vi "Process.vi"(8 "error in":errorcluster, 11 "Transport":refnum<class "SMO.Transport.lvclass">) -> (0 "error out":errorcluster, 3 "Transport out":refnum<class "SMO.Transport.lvclass">)   [LabVIEW 2019, in "SMO.Transport.lvclass"]
doc: "---------------------------------------------------------------\nJKI State Machine Objects™\nhttp://jki.net/state-machine-objects/\nCopyright (C) 2005-2015, JKI <info@jki.net>\nALL RIGHTS RESERVED"
uses:
  SMO.Transport.lvclass
  C:/Program Files (x86)/National Instruments/LabVIEW 2019/vi.lib/JKI/JKI SMO/SMO/SMO.lvclass
  SMO.Transport.lvclass/SMO.Transport.ctl
  Transport/Transport.lvclass/Transport.ctl
  <vilib>/JKI/JKI SMO/SMO/SMO.lvclass/SMO.ctl
  <userlib>/LevyLab/Instrument Framework/Instrument Types/Cryostat/Typedefs/Magnet Axis--Enum.ctl
  <userlib>/LevyLab/Instrument Framework/Instrument Types/Cryostat/Typedefs/Magnet Mode--Enum.ctl
  <userlib>/LevyLab/Lockin-Multichannel/Instrument.DAQ/Typedefs/Sweep.Configuration--Cluster.ctl
  <userlib>/LevyLab/Lockin-Multichannel/Instrument.DAQ/Typedefs/Sweep.Channel--Cluster--Array.ctl
  <userlib>/LevyLab/Lockin-Multichannel/Instrument.DAQ/Typedefs/Sweep.Channel--Cluster.ctl
  <userlib>/LevyLab/Lockin-Multichannel/Instrument.DAQ/Typedefs/Sweep.Pattern--Enum.ctl
  <vilib>/JKI/JKI SMO/SMO/Private/ReftoDVR--SMO.vi
  Control Experiment/Control Experiment.lvclass
  <vilib>/JKI/JKI SMO/SMO/SMO.lvclass
  <userlib>/LevyLab/Instrument Framework/Instrument Types/Cryostat/Instrument.Cryostat.lvclass
  <userlib>/LevyLab/Instrument Framework/Instrument Types/Strain/Instrument.Strain.lvclass
  <userlib>/LevyLab/Instrument Framework/Instrument Types/Delay Line/Instrument.DelayLine.lvclass
  <userlib>/LevyLab/Instrument Framework/Instrument Types/CBridge/Instrument.CBridge.lvclass
  <userlib>/LevyLab/Lockin-Multichannel/Instrument.Lockin/Instrument.Lockin.lvclass
  Transport/Transport.lvclass
  <userlib>/LevyLab/Lockin-Multichannel/Instrument.DAQ/Instrument.DAQ.lvclass
panel:
  # "For instructions on how to use the JKI State Machine Objects, examples and video tutorials, visit:\nhttp://jki.net/state-machine-objects/\n\nJKI State Machine Objects™\nhttp://jki.net/state-machine-objects/\nCopyright (C) 2005-2015, JKI <info@jki.net>\nALL RIGHTS RESERVED"
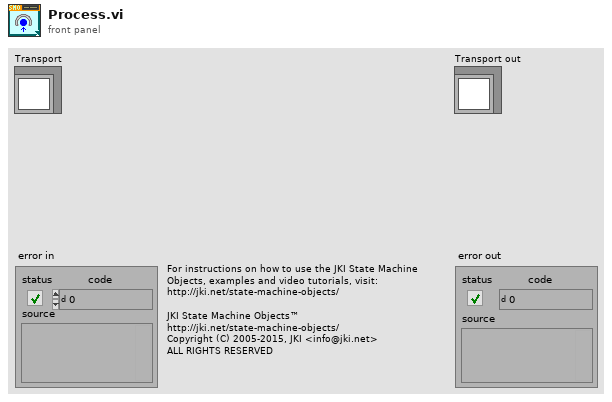
[diagram p1: front panel]
types:
  T1 = enum32{"invalid app kind", "Development System", "Run Time System", "Student Edition", "Embedded LabVIEW", "Evaluation", "Custom"}
  T2 = enum32{"Invalid", "Standard", "Closed", "Hidden", "Minimized", "Maximized"}
  T3 = enum32{"Bad", "Idle", "Run top level", "Running"}
  T4 = typedef "Instrument.Cryostat.lvclass/Magnet Mode--Enum.ctl" = enum16{"Persistent", "Driven"}
  T5 = typedef "Instrument.Cryostat.lvclass/Magnet Axis--Enum.ctl" = enum16{"Z", "X", "Y"}
  T6 = typedef "Instrument.DAQ.lvclass/Sweep.Configuration--Cluster.ctl" = cluster{"Sweep Time (s)":dbl, "Initial Wait (s)":dbl, "Return to Start":bool, "Channels":T7}
  T7 = typedef "Instrument.DAQ.lvclass/Sweep.Channel--Cluster--Array.ctl" = T8[]
  T8 = typedef "Instrument.DAQ.lvclass/Sweep.Channel--Cluster.ctl" = cluster{"Enable?":bool, "Channel":u16, "Start":dbl, "End":dbl, "Pattern":T9, "Table":dbl[]}
  T9 = typedef "Instrument.DAQ.lvclass/Sweep.Pattern--Enum.ctl" = enum16{"Ramp /", "Ramp /\\", "Smooth Ramp _/", "Smooth Ramp _/\\_", "Table"}
  T10 = typedef "Control Experiment.lvclass/Instruments--cluster.ctl" = cluster{"KH7008":refnum<class "Instrument.KH7008.lvclass">[], "Lockin":refnum<class "Instrument.Lockin.lvclass">, "Temperature":refnum<class "Instrument.Cryostat.lvclass">, "Magnet":refnum<class "Instrument.Cryostat.lvclass">, "Rotator":refnum<class "Instrument.Cryostat.lvclass">, "Level":refnum<class "Instrument.Cryostat.lvclass">, "Capacitance Bridge":refnum<class "Instrument.CBridge.lvclass">, "Delay Line":refnum<class "Instrument.DelayLine.lvclass">, "Strain Cell":refnum<class "Instrument.Strain.lvclass">, "VNA":refnum<class "Instrument.VNA.lvclass">, "Voltage Source":refnum<class "Instrument.VSource.lvclass">}
  T11 = cluster{"Core":cluster{"Current VI Reference":refnum<vi>, "Close Panel on Exit?":bool, "error":errorcluster}, "Self Reference":refnum<class "SMO.Transport.lvclass">, "C.E.":refnum<class "Control Experiment.lvclass">, "Instruments":T10, "value":variant, "wait":bool}
  T12 = cluster{"Current VI Reference":refnum<vi>, "Close Panel on Exit?":bool, "error":errorcluster}
  T13 = typedef "SMO.lvclass/Protected Events.ctl" = cluster{"StopProcesses":refnum<user-event>, "AbortProcesses":refnum<user-event>, "Config Changed":refnum<user-event>, "Dependency":refnum<user-event>}
  T14 = typedef "SMO.Transport.lvclass/PrivateEvents--Cluster.ctl" = cluster{"Configure":refnum<user-event>}
  T15 = typedef "Instrument.DAQ.lvclass/Get State-enum.ctl" = enum16{"idle", "created", "started", "stopped", "sweeping"}
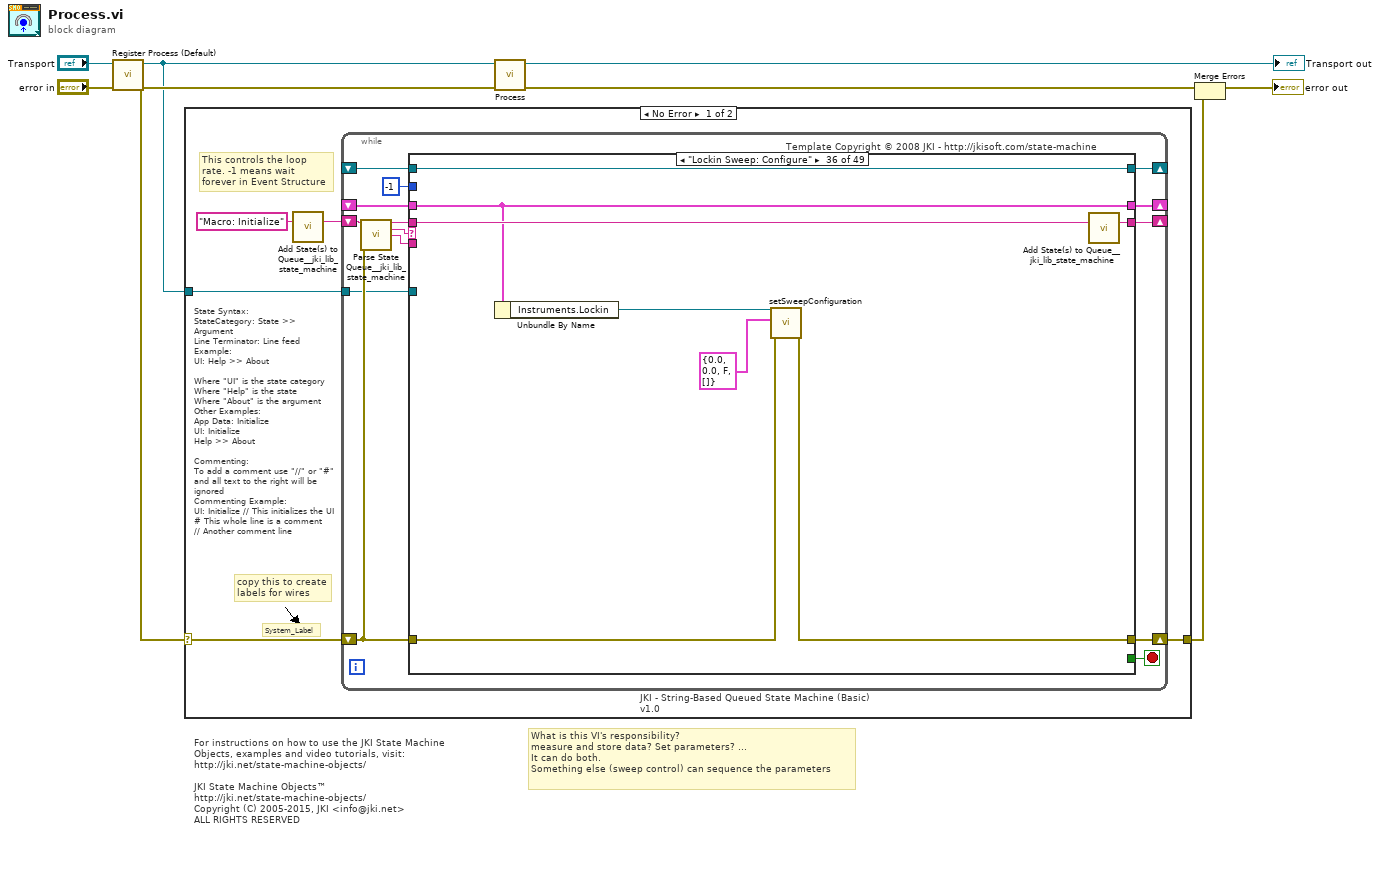
[diagram p0: block diagram]
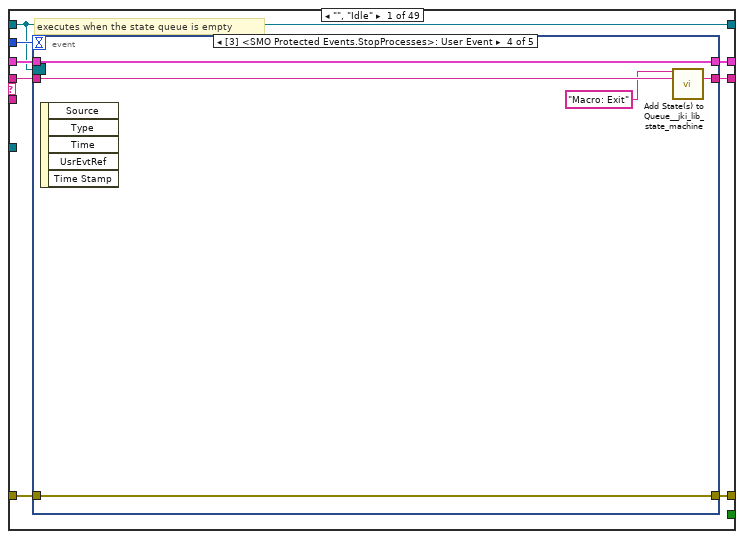
[diagram p2: hidden frame]
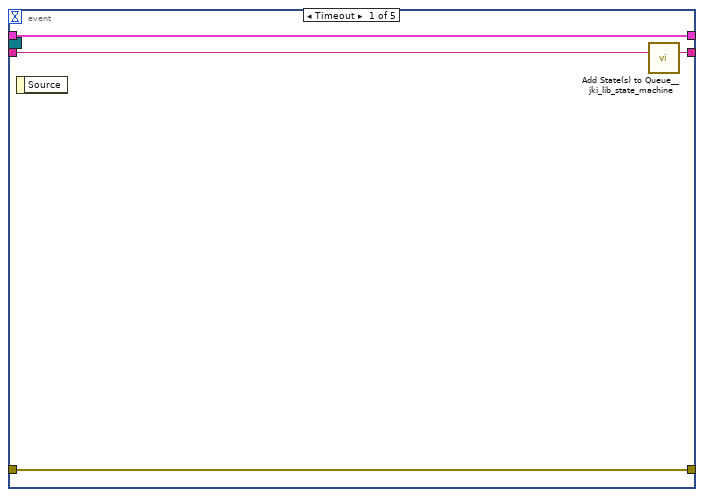
[diagram p3: hidden frame]
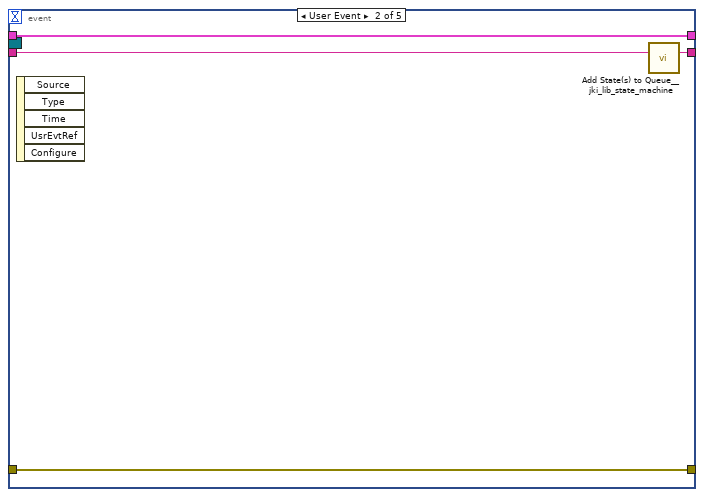
[diagram p4: hidden frame]
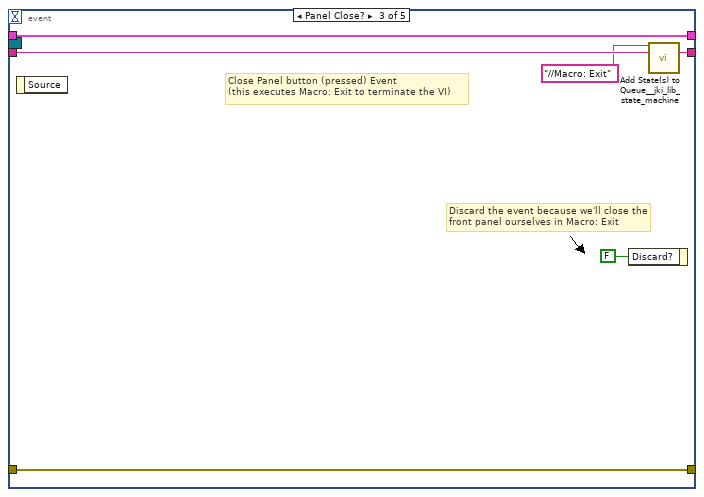
[diagram p5: hidden frame]
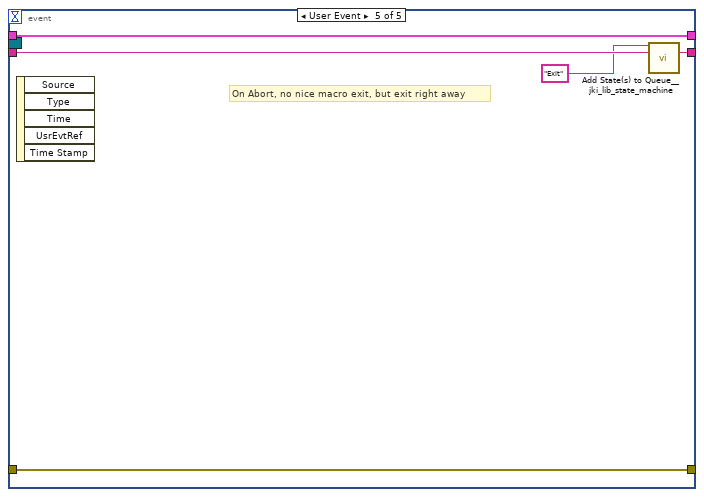
[diagram p6: hidden frame]
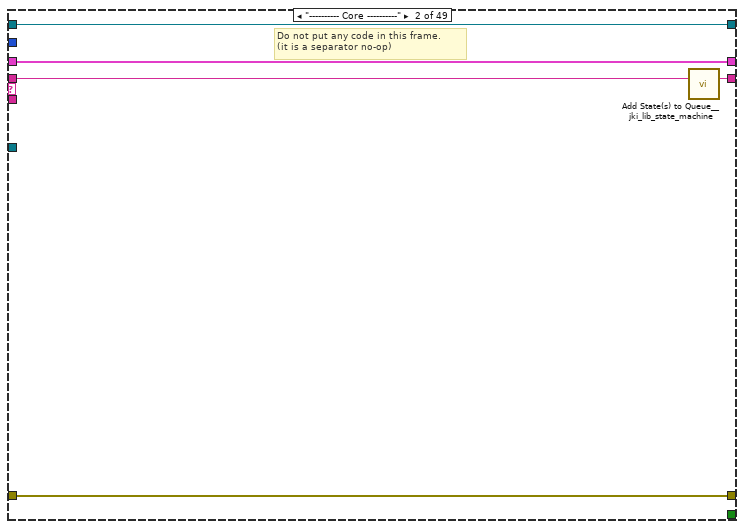
[diagram p7: hidden frame]
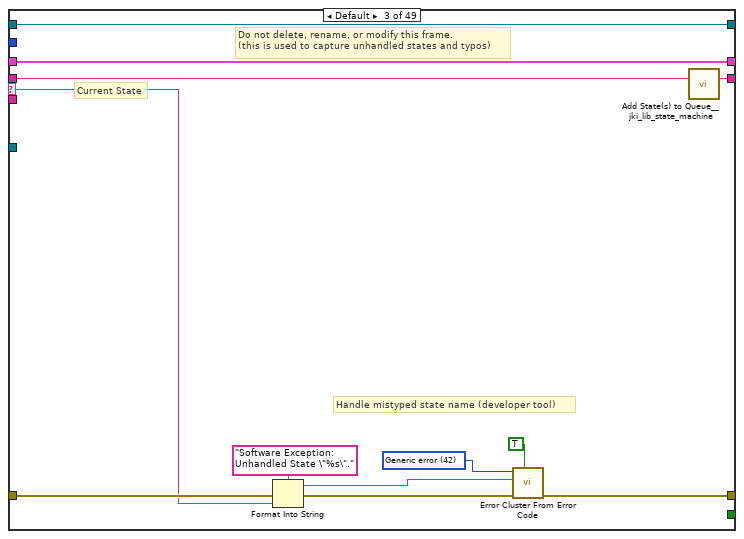
[diagram p8: hidden frame]
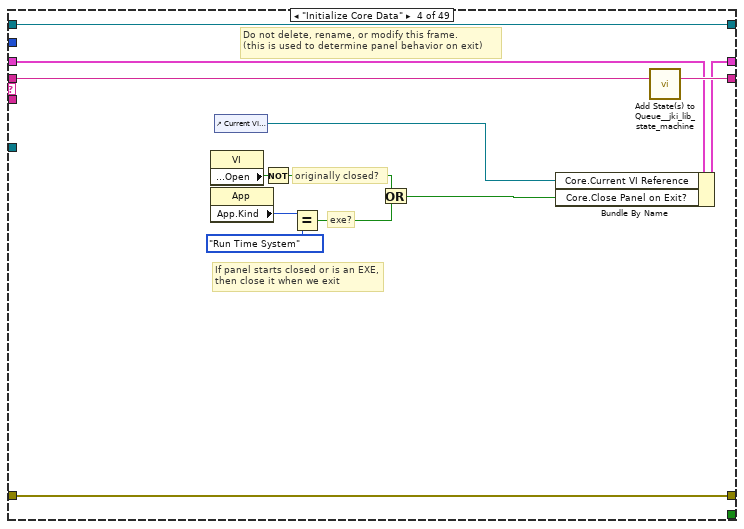
[diagram p9: hidden frame]
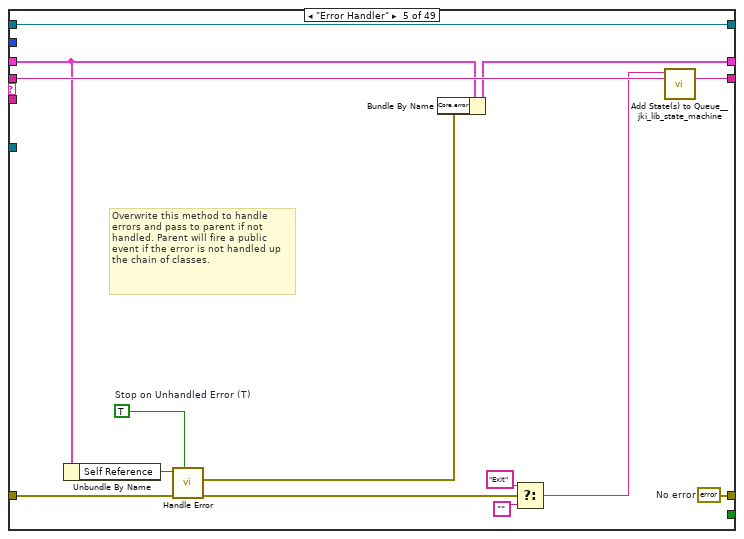
[diagram p10: hidden frame]
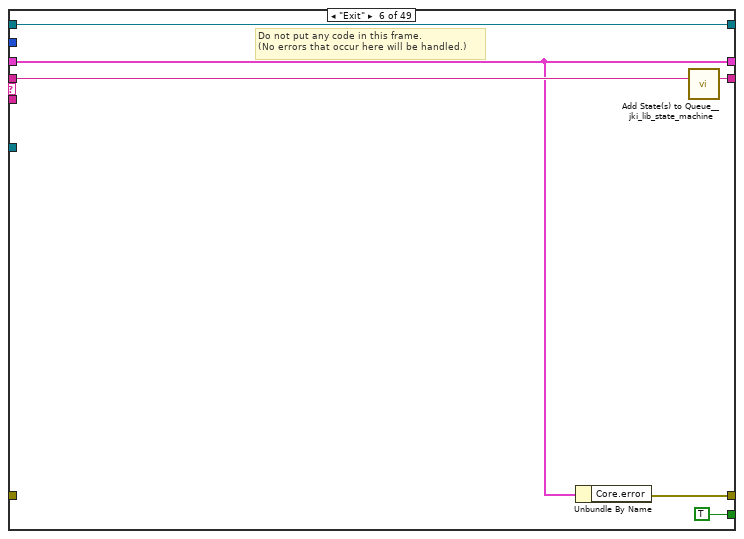
[diagram p11: hidden frame]
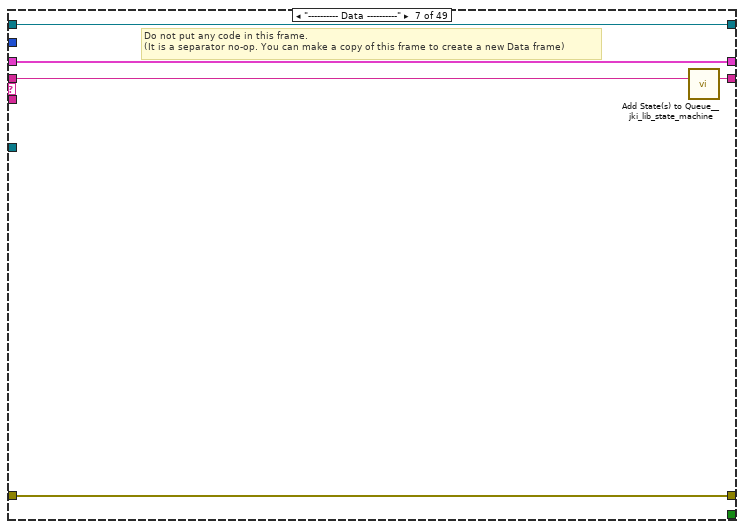
[diagram p12: hidden frame]
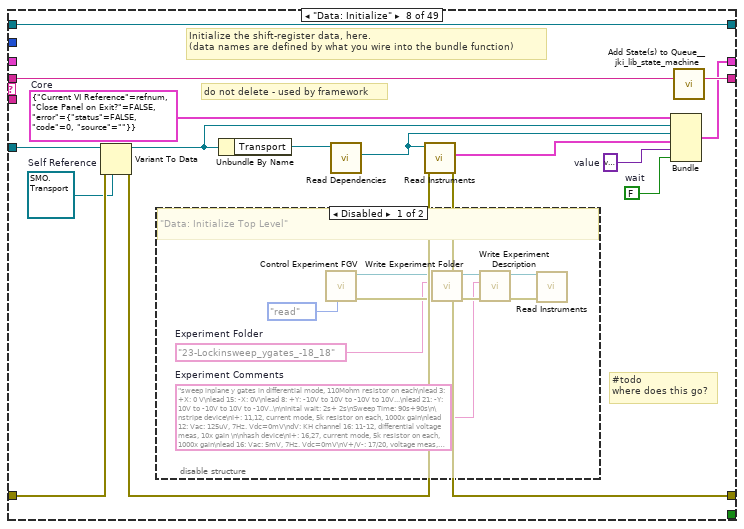
[diagram p13: hidden frame]
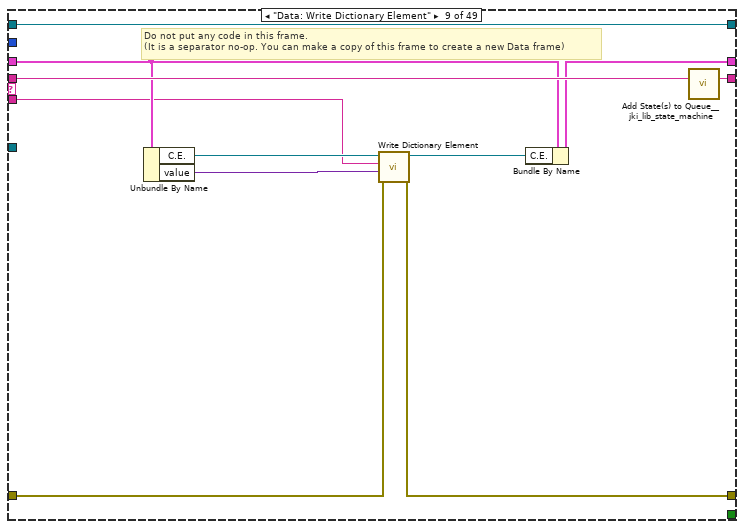
[diagram p15: hidden frame]
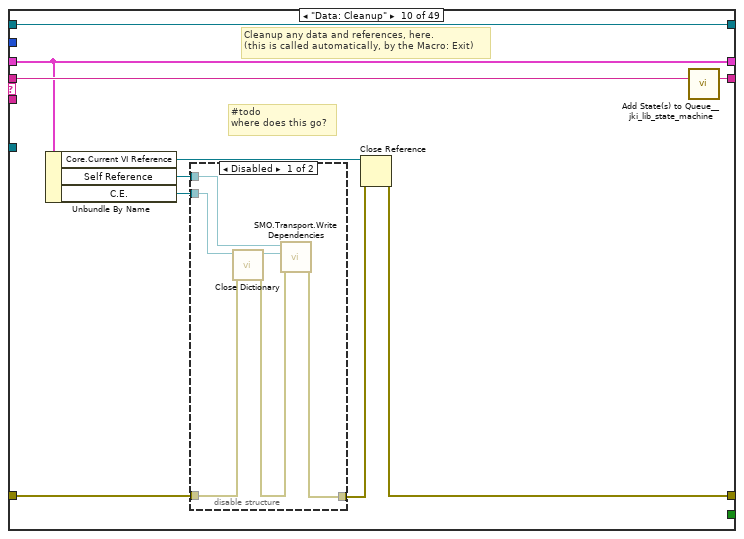
[diagram p16: hidden frame]
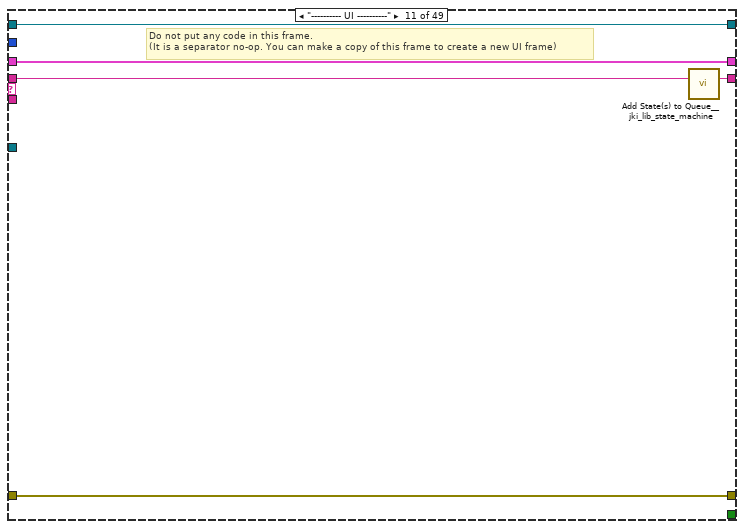
[diagram p18: hidden frame]
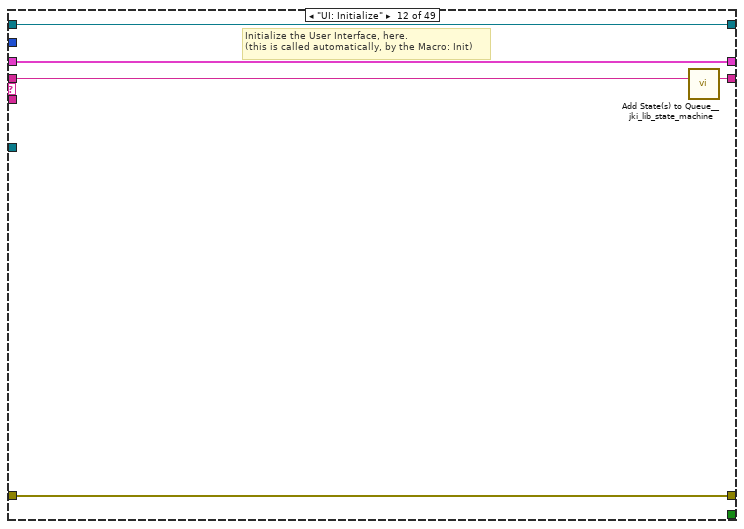
[diagram p19: hidden frame]
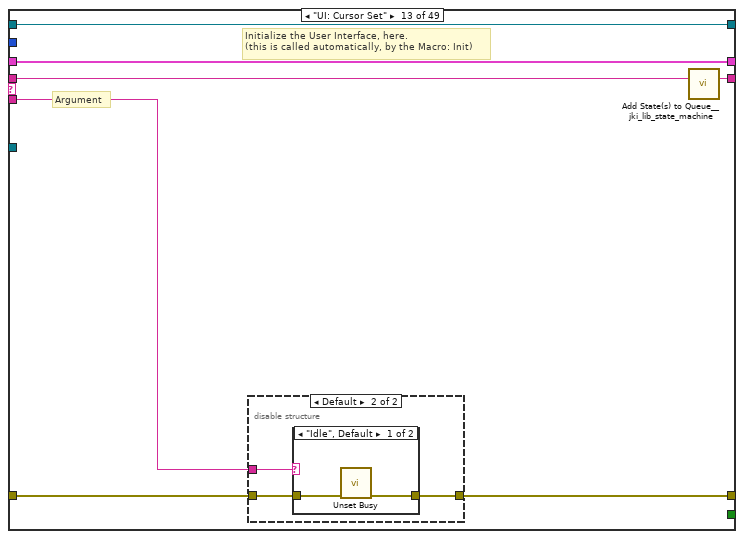
[diagram p20: hidden frame]
diagram:
  # "What is this VI's responsibility?\nmeasure and store data? Set parameters? ...\nIt can do both.\nSomething else (sweep control) can sequence the parameters"
  # "For instructions on how to use the JKI State Machine Objects, examples and video tutorials, visit:\nhttp://jki.net/state-machine-objects/\n\nJKI State Machine Objects™\nhttp://jki.net/state-machine-objects/\nCopyright (C) 2005-2015, JKI <info@jki.net>\nALL RIGHTS RESERVED"
  n1 = call <vilib>:"Register Process (Default).vi"("error in (no error)"="error in", "SMO"="Transport") -> ("error out"=w5:errorcluster, "SelfRef"=w4:refnum<class "SMO.Transport.lvclass">)  [unwired: 8 in]
  n2 = case shown="No Error" w5 {
    selector: w5 -> [w10 w561]
    tunnel: w4 -> [w11 _]
    tunnel: [w9 w561] -> w1
    frame No Error {
      # "State Syntax:\nStateCategory: State >> Argument\nLine Terminator: Line feed\nExample:\nUI: Help >> About\n\nWhere \"UI\" is the state category\nWhere \"Help\" is the state\nWhere \"About\" is the argument\nOther Examples:\nApp Data: Initialize\nUI: Initialize\nHelp >> About\n\nCommenting:\nTo add a comment use \"//\" or \"#\" and all text to the right will be ignored\nCommenting Example:\nUI: Initialize // This initializes the UI\n# This whole line is a comment\n// Another comment line"
      # "copy this to create labels for wires"
      # "This controls the loop rate. -1 means wait forever in Event Structure"
      # "System_Label"
      n3 = call <vilib>:"Add State(s) to Queue__jki_lib_state_machine.vi"("State(s) in (\"\")"="Macro: Initialize") -> ("States Out"=w13:string)  [unwired: 14 in]
      n4 = while "JKI - String-Based Queued State Machine (Basic) v1.0" {
        shift-right: [w20] -> _
        shift-left: _ -> [w19]
        shift-right: [w23] -> w9
        shift-left: w10 -> [w17]
        shift-right: [w22] -> _
        shift-left: w13 -> [w24]
        tunnel: w11 -> [w16]
        shift-right: [w15] -> _
        shift-left: _ -> [w14]
        stop <- w21 stop-if-true
        # "Template Copyright © 2008 JKI - http://jkisoft.com/state-machine"
        n5 = call <vilib>:"Parse State Queue__jki_lib_state_machine.vi"("State Queue"=w24, "Error In (no error)"=w17) -> ("Remaining States"=w26:string, "Current State"=w27:string, "Arguments"=w25:string)  [unwired: 11 in]
        n6 = case shown="\"Lockin Sweep: Configure\"" w27 {
          selector: w27 -> [_ _ w66 _ _ _ _ _ _ _ _ _ _ _ _ _ _ _ _ _ _ _ _ _ w312 _ _ _ _ _ _ _ _ _ _ _ _ _ _ _ _ _ _ _ _ _ _ _ _]
          tunnel: w26 -> [w35 w64 w70 w89 w103 w109 w114 w130 w150 w160 w172 w177 w184 w200 w232 w246 w251 w265 w270 w281 w286 w298 w304 w309 w324 w334 w348 w362 w374 w386 w398 w410 w422 w434 w441 w449 w458 w467 w475 w480 w488 w497 w506 w515 w524 w533 w542 w551 w560]
          tunnel: w25 -> [_ _ _ _ _ _ _ _ w140 _ _ _ w178 w194 _ _ _ _ _ _ _ _ _ _ w313 w325 w343 w357 w369 w381 w393 w405 w417 w429 _ _ _ _ _ _ _ _ _ _ _ _ _ _ _]
          tunnel: w19 -> [w33 w61 w68 w80 w97 w105 w111 _ w145 w151 w169 w175 w182 w196 w229 w242 w248 w256 w267 w278 w283 w296 w302 w306 w320 w330 w344 w358 w370 w382 w394 w406 w418 w430 w438 w446 w455 w464 w472 w478 w485 w491 w500 w509 w518 w527 w536 w545 w554]
          tunnel: [w32 w62 w72 w86 w98 w104 w112 w119 w142 w157 w170 w174 w179 w197 w230 w244 w249 w263 w268 w272 w284 w292 w300 w307 w322 w331 w345 w359 w371 w383 w395 w407 w419 w431 w439 w443 w450 w459 w469 w476 w482 w493 w502 w511 w520 w529 w538 w547 w556] -> w23
          tunnel: w17 -> [w31 w62 w71 w86 w99 _ w112 w127 w143 w153 w170 w174 w180 w198 w230 w244 w249 w263 w268 w273 w284 w293 w300 w307 w322 w326 w337 w353 w365 w377 w389 w401 w413 w425 w439 w444 w453 w462 w470 w476 w482 w489 w498 w507 w516 w525 w534 w543 w552]
          tunnel: [w34 w63 w69 w88 w102 w108 w113 w129 w149 w159 w171 w176 w183 w199 w231 w245 w250 w264 w269 w280 w285 w297 w303 w308 w323 w333 w347 w361 w373 w385 w397 w409 w421 w433 w440 w448 w457 w466 w474 w479 w487 w496 w505 w514 w523 w532 w541 w550 w559] -> w22
          tunnel: [_ _ _ _ _ TRUE _ _ _ _ _ _ _ _ _ _ _ _ _ _ _ _ _ _ _ _ _ _ _ _ _ _ _ _ _ _ _ _ _ _ _ _ _ _ _ _ _ _ _] -> w21
          tunnel: [w30 w61 w68 w87 w96 w105 w111 w128 w144 w151 w169 w175 w182 w196 w229 w242 w248 w256 w267 w278 w283 w296 w302 w306 w319 w330 w344 w358 w370 w382 w394 w406 w418 w430 w438 w446 w455 w464 w472 w478 w484 w494 w503 w512 w521 w530 w539 w548 w557] -> w20
          tunnel: -1 ("Timeout") -> [w29 _ _ _ _ _ _ _ _ _ _ _ _ _ _ _ _ _ _ _ _ _ _ _ _ _ _ _ _ _ _ _ _ _ _ _ _ _ _ _ _ _ _ _ _ _ _ _ _]
          tunnel: w16 -> [_ _ _ _ _ _ _ w126 _ _ _ _ _ _ _ _ _ _ _ _ _ _ _ _ _ _ _ _ _ _ _ _ _ _ _ _ _ _ _ _ _ _ _ _ _ _ _ _ _]
          tunnel: [w28 w60 w65 w77 w101 w106 w110 w125 w148 w156 w168 w173 w181 w193 w228 w243 w247 w257 w266 w279 w282 w295 w301 w305 w321 w332 w346 w360 w372 w384 w396 w408 w420 w432 w437 w447 w456 w465 w473 w477 w486 w495 w504 w513 w522 w531 w540 w549 w558] -> w15
          tunnel: w14 -> [w28 w60 w65 w77 w101 w106 w110 w125 w148 w156 w168 w173 w181 w193 w228 w243 w247 w257 w266 w279 w282 _ w301 w305 w321 w332 w346 w360 w372 w384 w396 w408 w420 w432 w437 w447 w456 w465 w473 w477 w486 w495 w504 w513 w522 w531 w540 w549 w558]
          frame "", "Idle" {
            # "executes when the state queue is empty"
            n7 = event shown="[3] <SMO Protected Events.StopProcesses>: User Event" {
              selector: w28 -> [_ _ _ _ _]
              dyn-events: _ -> [_ _ _ _ _]
              timeout: w29 -> [_ _ _ _ _]
              tunnel: w35 -> [w39 w43 w49 w54 w59]
              tunnel: [w38 w42 w48 w53 w58] -> w34
              tunnel: w33 -> [w37 w41 w46 w51 w56]
              tunnel: [w36 w40 w47 w52 w57] -> w32
              tunnel: w31 -> [w36 w40 w47 w52 w57]
              tunnel: [w37 w41 w46 w51 w56] -> w30
              event Timeout {
                n8 = event-data() -> ()  [unwired: 1 in, 1 out]
                n9 = call <vilib>:"Add State(s) to Queue__jki_lib_state_machine.vi"("State(s) in (\"\")"=w39) -> ("States Out"=w38:string)  [unwired: 14 in]
              }
              event User Event {
                n10 = event-data() -> ()  [unwired: 1 in, 5 out]
                n11 = call <vilib>:"Add State(s) to Queue__jki_lib_state_machine.vi"("State(s) in (\"\")"=w43) -> ("States Out"=w42:string)  [unwired: 14 in]
              }
              event Panel Close? {
                # "Discard the event because we'll close the front panel ourselves in Macro: Exit"
                # "Close Panel button (pressed) Event\n(this executes Macro: Exit to terminate the VI)"
                n12 = event-data() -> ()  [unwired: 1 in, 1 out]
                n13 = event-data("Discard?"=FALSE) -> ()  [unwired: 1 in, 1 out]
                n14 = call <vilib>:"Add State(s) to Queue__jki_lib_state_machine.vi"("State(s) in Front (\"\")"="//Macro: Exit", "State(s) in (\"\")"=w49) -> ("States Out"=w48:string)  [unwired: 13 in]
              }
              event User Event {
                n15 = event-data() -> ()  [unwired: 1 in, 5 out]
                n16 = call <vilib>:"Add State(s) to Queue__jki_lib_state_machine.vi"("State(s) in Front (\"\")"="Macro: Exit", "State(s) in (\"\")"=w54) -> ("States Out"=w53:string)  [unwired: 13 in]
              }
              event User Event {
                # "On Abort, no nice macro exit, but exit right away"
                n17 = event-data() -> ()  [unwired: 1 in, 5 out]
                n18 = call <vilib>:"Add State(s) to Queue__jki_lib_state_machine.vi"("State(s) in Front (\"\")"="Exit", "State(s) in (\"\")"=w59) -> ("States Out"=w58:string)  [unwired: 13 in]
              }
            }
          }
          frame "---------- Core ----------" {
            # "Do not put any code in this frame.\n(it is a separator no-op)"
            n19 = call <vilib>:"Add State(s) to Queue__jki_lib_state_machine.vi"("State(s) in (\"\")"=w64) -> ("States Out"=w63:string)  [unwired: 14 in]
          }
          frame Default {
            w75 = 42 items=["No error", "Argument error", "Memory is full", "Out of zone", "End of file", "File already open", "Generic file I/O error", "File not found", "File permission error", "Disk is full", "Duplicate path", "Too many files open", "System feature not enabled", "Resource file not found", "Cannot add resource", "Resource not found", "Image not found", "Image memory error", "Pen does not exist", "Config type invalid", "Config token not found", "Config parse error", "Config memory error", "Bad external code format", "Bad external code offset", "External code not present", "Null window", "Destroy window error", "Null menu", "Print aborted", "Bad print record", "Print driver error", "Windows error during printing", "Memory error during printing", "Print dialog error", "Generic print error", "Invalid device refnum", "Device not found", "Device parameter error", "Device unit error", "Cannot open device", "Device call aborted", "Generic error", "Cancelled by user", "Object ID too low", "Object ID too high", "Object not in heap", "Unknown heap", "Unknown object (invalid DefProc)", "Unknown object (DefProc not in table)", "Message out of range", "Invalid (null) method", "Unknown message", "Manager call not supported", "Bad address", "Network operation in progress", "Network operation timed out", "Connection is busy", "Network attribute not supported", "Network error", "Address in use", "System out of memory", "Connection aborted", "Connection refused", "Not connected", "Already connected", "Connection closed", "Initialization error (interapplication manager)", "Bad occurrence", "Wait on unbound occurrence handler", "Occurrence queue overflow", "Datalog type conflict", "Unused", "Unrecognized type (interapplication manager)", "Memory corrupt", "Failed to make temporary DLL", "Old CIN version", "Drag socket not found", "Failed to load drop-object", "Failed to register OLE object", "Failed to release OLE object", "Format specifier type mismatch", "Unknown format specifier", "Too few format specifiers", "Too many format specifiers", "Scan failed", "Newer CIN version", "Error converting to variant", "Runtime menu error", "Password tampered", "Variant attribute not found", "Incompatible variant data type", "Event data is not available", "Event Store is not present", "Occurrence is not found", "Event Queue is not created", "Event info is not available", "Refnum passed is NULL", "Error retrieving Class GUID", "Error retrieving CoClass GUID", "Error retrieving TypeLib GUID.", "Bad built application magic bytes.", "Specific driver is different from the specific driver associated with the Logical Name.", "There is no session opened to the class driver.", "Max Error", "MAX - Error with config objects", "MAX - Error loading configuration", "MAX - Group not supported"]
            # "Current State"
            # "Do not delete, rename, or modify this frame.\n(this is used to capture unhandled states and typos)"
            # "Handle mistyped state name (developer tool)"
            n20 = Format Into String(format string="Software Exception: Unhandled State \"%s\"." ("message"), error in=w71, w66) -> (resulting string=w74:string, error out=w73:errorcluster)  [unwired: 1 in]
            n21 = call <vilib>:"Error Cluster From Error Code.vi"("show call chain? (False)"=TRUE, "error in (no error)"=w73, "error message (\"\")"=w74, "error code (0)"=w75) -> ("error out"=w72:errorcluster)  [unwired: 5 in]
            n22 = call <vilib>:"Add State(s) to Queue__jki_lib_state_machine.vi"("State(s) in (\"\")"=w70) -> ("States Out"=w69:string)  [unwired: 14 in]
          }
          frame "Initialize Core Data" {
            # "Do not delete, rename, or modify this frame.\n(this is used to determine panel behavior on exit)"
            # "originally closed?"
            # "exe?"
            # "If panel starts closed or is an EXE, then close it when we exit"
            n23 = property class="VI"() -> ("Front Panel.Open"=w85:bool)  [unwired: 2 in, 2 out]
            n24 = property class="App"() -> ("App.Kind"=w84:T1)  [unwired: 2 in, 2 out]
            n25 = control-ref of="Current VI Reference"() -> (w78:refnum<vi>)
            n26 = Not(x=w85) -> (.not. x?=w82:bool)
            n27 = Equal?(x=w84, y=T1."Run Time System" ("Application:Kind")) -> (x = y?=w81:bool)
            n28 = Or(x=w82, y=w81) -> (x .or. y?=w79:bool)
            n29 = Bundle By Name(cluster=w80, "Core.Current VI Reference"=w78, "Core.Close Panel on Exit?"=w79) -> (w87:T11)
            n30 = call <vilib>:"Add State(s) to Queue__jki_lib_state_machine.vi"("State(s) in (\"\")"=w89) -> ("States Out"=w88:string)  [unwired: 14 in]
          }
          frame "Error Handler" {
            w90 = TRUE  # Stop on Unhandled Error (T)
            w98 = errorcluster {"status"=FALSE, "code"=0, "source"=""}  # No error
            # "Overwrite this method to handle errors and pass to parent if not handled. Parent will fire a public event if the error is not handled up the chain of classes."
            n31 = Unbundle By Name(w97) -> ("Self Reference"=w100:refnum<class "SMO.Transport.lvclass">)
            n32 = call-dynamic "Handle Error.vi"("Stop on Unhandled Error (T)"=w90, "error in"=w99, "SMO"=w100) -> ("handling error"=w91:errorcluster, "Unhandled error"=w94:errorcluster)  [unwired: 6 in, 1 out]
            n33 = Bundle By Name(cluster=w97, "Core.error"=w94) -> (w96:T11)
            n34 = Select(t="Exit", s=w91, f="") -> (s? t:f=w95:string)
            n35 = call <vilib>:"Add State(s) to Queue__jki_lib_state_machine.vi"("State(s) in Front (\"\")"=w95, "State(s) in (\"\")"=w103) -> ("States Out"=w102:string)  [unwired: 13 in]
          }
          frame "Exit" {
            # "Do not put any code in this frame.\n(No errors that occur here will be handled.)"
            n36 = Unbundle By Name(w105) -> ("Core.error"=w104:errorcluster)
            n37 = call <vilib>:"Add State(s) to Queue__jki_lib_state_machine.vi"("State(s) in (\"\")"=w109) -> ("States Out"=w108:string)  [unwired: 14 in]
          }
          frame "---------- Data ----------" {
            # "Do not put any code in this frame.\n(It is a separator no-op. You can make a copy of this frame to create a new Data frame)"
            n38 = call <vilib>:"Add State(s) to Queue__jki_lib_state_machine.vi"("State(s) in (\"\")"=w114) -> ("States Out"=w113:string)  [unwired: 14 in]
          }
          frame "Data: Initialize" {
            w118 = FALSE  # wait
            w122 = variant  # value
            w123 = refnum<class "SMO.Transport.lvclass"> refnum  # Self Reference
            w124 = T12 {"Current VI Reference"=refnum, "Close Panel on Exit?"=FALSE, "error"={"status"=FALSE, "code"=0, "source"=""}}  # Core
            # "#todo\nwhere does this go?"
            # "do not delete - used by framework"
            # "Initialize the shift-register data, here.\n(data names are defined by what you wire into the bundle function)"
            n39 = Variant To Data(error in=w127, type=w123, Variant=w126) -> (data=w117:refnum<class "SMO.Transport.lvclass">, error out=w120:errorcluster)
            n40 = disable-structure shown="Disabled" {
              frame Disabled {
                w133 = "sweep inplane y gates in differential mode, 110Mohm resistor on each\nlead 3: +X: 0 V\nlead 15: -X: 0V\nlead 8: +Y: -10V to 10V to -10V to 10V...\nlead 21: -Y: 10V to -10V to 10V to -10V..\n\nInital wait: 2s+ 2s\nSweep Time: 90s+90s\n\nstripe device\nI+: 11,12, current mode, 5k resistor on each, 1000x gain\nlead 12: Vac: 125uV, 7Hz. Vdc=0mV\ndV: KH channel 16: 11-12, differential voltage meas, 10x gain \n\nhash device\nI+: 16,27, current mode, 5k resistor on each, 1000x gain\nlead 16: Vac: 5mV, 7Hz. Vdc=0mV\nV+/V-: 17/20, voltage meas, 10x gain \nKH 5: 17-20, volt. meas., 10x gain\n\n\nlead 26: Vbg: 0V, 1Gohm resistor\nB: -18T to 18T @0.033T/min\n"  # Experiment Comments
                w134 = "23-Lockinsweep_ygates_-18_18"  # Experiment Folder
                # "\"Data: Initialize Top Level\""
                n41 = call "Control Experiment FGV.vi"("Function"=enum16{"read", "write"}."read") -> ("error out"=w138:errorcluster, "Control Experiment.lvclass out"=w139:refnum<class "Control Experiment.lvclass">)  [unwired: 9 in]
                n42 = call "Write Experiment Folder.vi"("error in (no error)"=w138, "Experiment Folder"=w134, "Control Experiment in"=w139) -> ("error out"=w136:errorcluster, "Control Experiment out"=w137:refnum<class "Control Experiment.lvclass">)  [unwired: 7 in]
                n43 = call "Write Experiment Description.vi"("error in (no error)"=w136, "Experiment Description"=w133, "Control Experiment in"=w137) -> ("error out"=w131:errorcluster, "Control Experiment out"=w132:refnum<class "Control Experiment.lvclass">)  [unwired: 7 in]
                n44 = call "Read Instruments.vi"("error in (no error)"=w131, "Control Experiment in"=w132) -> ()  [unwired: 7 in, 3 out]
              }
              frame Enabled {
              }
            }
            n45 = Unbundle By Name(w117) -> ("Transport"=w116:refnum<class "Transport.lvclass">)
            n46 = call "Read Dependencies.vi"("Transport"=w116) -> ("C.E."=w115:refnum<class "Control Experiment.lvclass">)  [unwired: 8 in, 2 out]
            n47 = call "Read Instruments.vi"("error in (no error)"=w120, "Control Experiment in"=w115) -> ("error out"=w119:errorcluster, "Instruments"=w121:T10)  [unwired: 7 in, 1 out]
            n48 = Bundle("Core"=w124, "Self Reference"=w117, "C.E."=w115, "Instruments"=w121, "value"=w122, "wait"=w118) -> (w128:T11)  [unwired: 1 in]
            n49 = call <vilib>:"Add State(s) to Queue__jki_lib_state_machine.vi"("State(s) in (\"\")"=w130) -> ("States Out"=w129:string)  [unwired: 14 in]
          }
          frame "Data: Write Dictionary Element" {
            # "Do not put any code in this frame.\n(It is a separator no-op. You can make a copy of this frame to create a new Data frame)"
            n50 = Unbundle By Name(w145) -> ("C.E."=w147:refnum<class "Control Experiment.lvclass">, "value"=w141:variant)
            n51 = call "Write Dictionary Element.vi"("error in (no error)"=w143, "value"=w141, "key"=w140, "Control Experiment in"=w147) -> ("error out"=w142:errorcluster, "Control Experiment out"=w146:refnum<class "Control Experiment.lvclass">)  [unwired: 6 in]
            n52 = Bundle By Name(cluster=w145, "C.E."=w146) -> (w144:T11)
            n53 = call <vilib>:"Add State(s) to Queue__jki_lib_state_machine.vi"("State(s) in (\"\")"=w150) -> ("States Out"=w149:string)  [unwired: 14 in]
          }
          frame "Data: Cleanup" {
            # "#todo\nwhere does this go?"
            # "Cleanup any data and references, here.\n(this is called automatically, by the Macro: Exit)"
            n54 = Unbundle By Name(w151) -> ("Core.Current VI Reference"=w158:refnum<vi>, "Self Reference"=w155:refnum<class "SMO.Transport.lvclass">, "C.E."=w154:refnum<class "Control Experiment.lvclass">)
            n55 = disable-structure shown="Disabled" {
              disable-tunnel: w155 -> [w161 _]
              disable-tunnel: w154 -> [w162 _]
              disable-tunnel: w153 -> [w165 w167]
              disable-tunnel: [w163 w167] -> w152
              frame Disabled {
                n56 = call "Close Dictionary.vi"("error in (no error)"=w165, "Control Experiment in"=w162) -> ("error out"=w164:errorcluster, "Control Experiment out"=w166:refnum<class "Control Experiment.lvclass">)  [unwired: 8 in]
                n57 = call "SMO.Transport.Write Dependencies.vi"("error in (no error)"=w164, "Transport.lvclass"=w166, "Transport in"=w161) -> ("error out"=w163:errorcluster)  [unwired: 7 in, 1 out]
              }
              frame Enabled {
              }
            }
            n58 = Close Reference(reference=w158, error in (no error)=w152) -> (error out=w157:errorcluster)
            n59 = call <vilib>:"Add State(s) to Queue__jki_lib_state_machine.vi"("State(s) in (\"\")"=w160) -> ("States Out"=w159:string)  [unwired: 14 in]
          }
          frame "---------- UI ----------" {
            # "Do not put any code in this frame.\n(It is a separator no-op. You can make a copy of this frame to create a new UI frame)"
            n60 = call <vilib>:"Add State(s) to Queue__jki_lib_state_machine.vi"("State(s) in (\"\")"=w172) -> ("States Out"=w171:string)  [unwired: 14 in]
          }
          frame "UI: Initialize" {
            # "Initialize the User Interface, here.\n(this is called automatically, by the Macro: Init)"
            n61 = call <vilib>:"Add State(s) to Queue__jki_lib_state_machine.vi"("State(s) in (\"\")"=w177) -> ("States Out"=w176:string)  [unwired: 14 in]
          }
          frame "UI: Cursor Set" {
            # "Argument"
            # "Initialize the User Interface, here.\n(this is called automatically, by the Macro: Init)"
            n62 = disable-structure shown="Default" {
              disable-tunnel: w180 -> [w185 w188]
              disable-tunnel: [w185 w187] -> w179
              disable-tunnel: w178 -> [_ w186]
              frame condition #0 {
              }
              frame condition #1 (active) {
                n63 = case shown="\"Idle\", Default" w186 {
                  tunnel: w188 -> [w190 w192]
                  tunnel: [w189 w191] -> w187
                  frame "Idle", Default {
                    n64 = call <vilib>:"Unset Busy.vi"("error in (no error)"=w190) -> ("error out"=w189:errorcluster)  [unwired: 10 in]
                  }
                  frame "Busy" {
                    n65 = call <vilib>:"Set Busy.vi"("error in (no error)"=w192) -> ("error out"=w191:errorcluster)  [unwired: 9 in, 1 out]
                  }
                }
              }
            }
            n66 = call <vilib>:"Add State(s) to Queue__jki_lib_state_machine.vi"("State(s) in (\"\")"=w184) -> ("States Out"=w183:string)  [unwired: 14 in]
          }
          frame "UI: Front Panel State" {
            # "Argument"
            # "Set Front Panel Open or Closed\n(Usage: \"UI: Front Panel State >> Open|Close\")"
            n67 = Unbundle By Name(w196) -> ("Core.Current VI Reference"=w195:refnum<vi>)
            n68 = disable-structure shown="Default" {
              disable-tunnel: w198 -> [w204 w227]
              disable-tunnel: [w203 w227] -> w197
              disable-tunnel: w195 -> [w202 _]
              disable-tunnel: w194 -> [w201 _]
              frame condition #0 (active) {
                n69 = case shown="\"Close\"" w201 {
                  tunnel: w204 -> [w208 w221]
                  tunnel: [w210 w222] -> w203
                  tunnel: w202 -> [w209 w219]
                  frame "Open", Default {
                    n70 = property class="VI"(reference=w209, error in=w208) -> (reference out=w206:refnum<vi>, error out=w207:errorcluster, "FP.State"=w205:T2)
                    n71 = case shown="\"Closed\"" w205 {
                      tunnel: [w213 w216] -> w210
                      tunnel: w207 -> [w212 w216]
                      tunnel: w206 -> [w211 _]
                      frame "Closed" {
                        n72 = invoke class="VI" method="FP.Open"(reference=w211, error in=w212, "Activate"=TRUE, "State"=T2."Standard") -> (error out=w213:errorcluster)  [unwired: 1 in, 4 out]
                      }
                      frame Default {
                      }
                    }
                  }
                  frame "Close" {
                    n73 = property class="VI"(reference=w219, error in=w221) -> (reference out=w218:refnum<vi>, error out=w220:errorcluster, "FP.State"=w217:T2)
                    n74 = case shown="Default" w217 {
                      tunnel: [w223 w226] -> w222
                      tunnel: w220 -> [w223 w225]
                      tunnel: w218 -> [_ w224]
                      frame "Invalid", "Closed" {
                      }
                      frame Default {
                        n75 = invoke class="VI" method="FP.Close"(reference=w224, error in=w225) -> (error out=w226:errorcluster)  [unwired: 1 in, 2 out]
                      }
                    }
                  }
                }
              }
              frame condition #1 {
              }
            }
            n76 = call <vilib>:"Add State(s) to Queue__jki_lib_state_machine.vi"("State(s) in (\"\")"=w200) -> ("States Out"=w199:string)  [unwired: 14 in]
          }
          frame "---------- Macro ----------" {
            # "Do not put any code in this frame.\n(It is a separator no-op. You can make a copy of this frame to create a new Macro frame)"
            n77 = call <vilib>:"Add State(s) to Queue__jki_lib_state_machine.vi"("State(s) in (\"\")"=w232) -> ("States Out"=w231:string)  [unwired: 14 in]
          }
          frame "Macro: Initialize" {
            w237 = "//UI: Initialize\n//UI: Front Panel State >> Open"  # //UI: Initialize //UI: Front Panel State >> Open
            w233 = "Process: Sync"
            # "Initialization Macro\n(This is called once, when the VI starts)"
            n78 = control-ref of="This VI"() -> (w235:refnum<vi>)
            n79 = property class="VI"(reference=w235) -> ("Exec.State"=w234:T3)  [unwired: 1 in, 2 out]
            n80 = Equal?(x=w234, y=T3."Run top level") -> (x = y?=w240:bool)
            n81 = Select(t=w233, s=w240, f="") -> ()  [unwired: 1 out]
            n82 = call <vilib>:"Add State(s) to Queue__jki_lib_state_machine.vi"("State(s) in Front (\"\")"="Data: Initialize\nInitialize Core Data\nEvents: Register", "State(s) in (\"\")"=w233, "State(s) at Back (\"\")"=w237) -> ("States Out"=w236:string)  [unwired: 12 in]
            n83 = call <vilib>:"Add State(s) to Queue__jki_lib_state_machine.vi"("State(s) in Front (\"\")"=w236, "State(s) in (\"\")"=w246) -> ("States Out"=w245:string)  [unwired: 13 in]
          }
          frame "Macro: Experiments" {
            # "Experimental Macros:\n- IV\n- Lockin_time\n- Lockin_Vsg\n- Lockin_sweep\n- Lockin_AIWFM_time\n- Sweep_AIWFM_time \n- Lockin?\n- THz_TimeDelay"
            # "Macro: Experiments\n(Placeholder for experiment macros)"
            n84 = call <vilib>:"Add State(s) to Queue__jki_lib_state_machine.vi"("State(s) in (\"\")"=w251) -> ("States Out"=w250:string)  [unwired: 14 in]
          }
          frame "Macro: Exit" {
            # "Exit Macro\n(This is called once, when the VI exits)"
            n85 = Unbundle By Name(w256) -> ("Core.Close Panel on Exit?"=w262:bool)
            n86 = Select(t="UI: Front Panel State >> Close", s=w262, f="") -> (s? t:f=w259:string)
            n87 = call <vilib>:"Add State(s) to Queue__jki_lib_state_machine.vi"("State(s) in Front (\"\")"="Data: Cleanup\nEvents: Unregister", "State(s) in (\"\")"="Process: Sync", "State(s) at Back (\"\")"="Exit") -> ("States Out"=w253:string)  [unwired: 12 in]
            n88 = call <vilib>:"Add State(s) to Queue__jki_lib_state_machine.vi"("State(s) in (\"\")"=w259, "State(s) at Back (\"\")"=w253) -> ("States Out"=w258:string)  [unwired: 13 in]
            n89 = call <vilib>:"Add State(s) to Queue__jki_lib_state_machine.vi"("State(s) in Front (\"\")"=w258, "State(s) in (\"\")"=w265) -> ("States Out"=w264:string)  [unwired: 13 in]
          }
          frame "---------- Process ----------" {
            # "Template Separator\n(You can make a copy of, or modify, this frame)"
            n90 = call <vilib>:"Add State(s) to Queue__jki_lib_state_machine.vi"("State(s) in (\"\")"=w270) -> ("States Out"=w269:string)  [unwired: 14 in]
          }
          frame "Process: Sync" {
            n91 = Unbundle By Name(w278) -> ("Self Reference"=w274:refnum<class "SMO.Transport.lvclass">)
            n92 = call <vilib>:"WaitOnProcessSync.vi"("error in (no error)"=w273, "SMO"=w274) -> ("error out"=w272:errorcluster, "Don't run?"=w277:bool)  [unwired: 7 in, 1 out]
            n93 = Select(t="Data: Cleanup\nEvents: Unregister\nExit", s=w277, f="") -> (s? t:f=w271:string)
            n94 = call <vilib>:"Add State(s) to Queue__jki_lib_state_machine.vi"("State(s) in Front (\"\")"=w271, "State(s) in (\"\")"=w281) -> ("States Out"=w280:string)  [unwired: 13 in]
          }
          frame "---------- Events ----------" {
            # "Template Separator\n(You can make a copy of, or modify, this frame)"
            n95 = call <vilib>:"Add State(s) to Queue__jki_lib_state_machine.vi"("State(s) in (\"\")"=w286) -> ("States Out"=w285:string)  [unwired: 14 in]
          }
          frame "Events: Register" {
            # "Expand to add\nmore events"
            n96 = Unbundle By Name(w296) -> ("Self Reference"=w289:refnum<class "SMO.Transport.lvclass">)
            n97 = call <vilib>:"GetProtectedEvents.vi"("SMO"=w289) -> ("error out"=w290:errorcluster, "SMO Protected Events"=w294:T13)  [unwired: 8 in, 1 out]
            n98 = call "SMO.Transport.GetPrivateEvents.vi"("Transport"=w289) -> ("error out"=w287:errorcluster, "Private Events"=w288:T14)  [unwired: 8 in, 1 out]
            n99 = register-events(w294, w288) -> (reference out=w295:refnum<event-registration>, error out=w291:errorcluster)  [unwired: 2 in]
            n100 = Merge Errors(w287, w293, w291, w290) -> (w292:errorcluster)
            n101 = call <vilib>:"Add State(s) to Queue__jki_lib_state_machine.vi"("State(s) in (\"\")"=w298) -> ("States Out"=w297:string)  [unwired: 14 in]
          }
          frame "Events: Unregister" {
            n102 = Unregister For Events(event registration refnum=w301, error in=w300) -> (error out=w299:errorcluster)
            n103 = call <vilib>:"Clear Errors.vi"("error in (no error)"=w299) -> ()  [unwired: 5 in, 2 out]
            n104 = call <vilib>:"Add State(s) to Queue__jki_lib_state_machine.vi"("State(s) in (\"\")"=w304) -> ("States Out"=w303:string)  [unwired: 14 in]
          }
          frame "---------- Set ----------" {
            n105 = call <vilib>:"Add State(s) to Queue__jki_lib_state_machine.vi"("State(s) in (\"\")"=w309) -> ("States Out"=w308:string)  [unwired: 14 in]
          }
          frame "Set: Wait" {
            # "#todo\nadd comments"
            n106 = Unbundle By Name(w320) -> ("wait"=w317:bool)
            n107 = call "Wait SubVI.vi"("time (ms)"=w313, "waiting"=w317) -> ("keep waiting"=w316:bool)  [unwired: 8 in, 1 out]
            n108 = call <vilib>:"Build State String with Arguments__JKI_lib_State_Machine.vi"("Arguments (\"\")"=w313, "State"=w312) -> ("State with Arguments"=w311:string)  [unwired: 4 in]
            n109 = call <vilib>:"Add State(s) to Queue__jki_lib_state_machine.vi"("State(s) in Front (\"\")"="Idle" ("format string"), "State(s) at Back (\"\")"=w311) -> ("States Out"=w310:string)  [unwired: 13 in]
            n110 = Bundle By Name(cluster=w320, "wait"=w316) -> (w319:T11)
            n111 = Select(t=w310, s=w316, f="") -> (s? t:f=w318:string)
            n112 = call <vilib>:"Add State(s) to Queue__jki_lib_state_machine.vi"("State(s) in Front (\"\")"=w318, "State(s) in (\"\")"=w324) -> ("States Out"=w323:string)  [unwired: 13 in]
          }
          frame "Set: Temperature" {
            # "#todo\nconvert string parm\nto data\n....JSON RPC?"
            n113 = Unbundle By Name(w330) -> ("Instruments.Temperature"=w327:refnum<class "Instrument.Cryostat.lvclass">)
            n114 = flat-sequence {
              tunnel: w325 -> [_]
              tunnel: [0.0 ("Target Field (T)")] -> w329
              tunnel: [0.0 ("Target Rate (T/min)")] -> w328
              frame #0 {
              }
            }
            n115 = call-dynamic "Set Temperature.vi"("error in (no error)"=w326, "Rate (K/min)"=w328, "Temperature (K)"=w329, "Instrument.Cryostat in"=w327) -> ("error out"=w331:errorcluster)  [unwired: 6 in, 1 out]
            n116 = call <vilib>:"Add State(s) to Queue__jki_lib_state_machine.vi"("State(s) in (\"\")"=w334) -> ("States Out"=w333:string)  [unwired: 14 in]
          }
          frame "Set: Magnet" {
            n117 = Unbundle By Name(w344) -> ("Instruments.Magnet"=w338:refnum<class "Instrument.Cryostat.lvclass">)
            n118 = flat-sequence {
              tunnel: w343 -> [_]
              tunnel: [0.0 ("Target Field (T)")] -> w342
              tunnel: [0.0 ("Target Rate (T/min)")] -> w341
              tunnel: [Magnet_Axis--Enum."Z" ("Axis")] -> w340
              tunnel: [Magnet_Mode--Enum."Persistent" ("Mode")] -> w339
              frame #0 {
              }
            }
            n119 = call-dynamic "Set Magnet.vi"("Mode"=w339, "Axis"=w340, "error in (no error)"=w337, "Target Rate (T/min)"=w341, "Target Field (T)"=w342, "Instrument.Cryostat in"=w338) -> ("error out"=w345:errorcluster)  [unwired: 4 in, 1 out]
            n120 = call <vilib>:"Add State(s) to Queue__jki_lib_state_machine.vi"("State(s) in (\"\")"=w348) -> ("States Out"=w347:string)  [unwired: 14 in]
          }
          frame "Set: Strain" {
            n121 = Unbundle By Name(w358) -> ("Instruments.Strain Cell"=w354:refnum<class "Instrument.Strain.lvclass">)
            n122 = flat-sequence {
              tunnel: w357 -> [_]
              tunnel: [0.0 ("Target Field (T)")] -> w356
              tunnel: [0.0 ("Target Rate (T/min)")] -> w355
              frame #0 {
              }
            }
            n123 = call-dynamic "Set Strain.vi"("error in (no error)"=w353, "Slew (V/s)"=w355, "Strain (V)"=w356, "Instrument.Strain in"=w354) -> ("error out"=w359:errorcluster)  [unwired: 6 in, 1 out]
            n124 = call <vilib>:"Add State(s) to Queue__jki_lib_state_machine.vi"("State(s) in (\"\")"=w362) -> ("States Out"=w361:string)  [unwired: 14 in]
          }
          frame "Set: Delay" {
            n125 = Unbundle By Name(w370) -> ("Instruments.Delay Line"=w366:refnum<class "Instrument.DelayLine.lvclass">)
            n126 = flat-sequence {
              tunnel: w369 -> [_]
              tunnel: [0.0 ("Target Field (T)")] -> w368
              tunnel: [0.0 ("Target Rate (T/min)")] -> w367
              frame #0 {
              }
            }
            n127 = call-dynamic "Set Delay.vi"("error in (no error)"=w365, "Rate (ps/s)"=w367, "Delay (ps)"=w368, "Instrument.Delay in"=w366) -> ("error out"=w371:errorcluster)  [unwired: 6 in, 1 out]
            n128 = call <vilib>:"Add State(s) to Queue__jki_lib_state_machine.vi"("State(s) in (\"\")"=w374) -> ("States Out"=w373:string)  [unwired: 14 in]
          }
          frame "Set: Lockin Channel Offset" {
            n129 = Unbundle By Name(w382) -> ("Instruments.Lockin"=w378:refnum<class "Instrument.Lockin.lvclass">)
            n130 = flat-sequence {
              tunnel: w381 -> [_]
              tunnel: [0 ("Target Field (T)")] -> w380
              tunnel: [0.0 ("Target Rate (T/min)")] -> w379
              frame #0 {
              }
            }
            n131 = call <userlib>:"setAO_DC.vi"("error in (no error)"=w377, "DC (V)"=w379, "AO Channel"=w380, "Instrument.Lockin in"=w378) -> ("error out"=w383:errorcluster)  [unwired: 6 in, 1 out]
            n132 = call <vilib>:"Add State(s) to Queue__jki_lib_state_machine.vi"("State(s) in (\"\")"=w386) -> ("States Out"=w385:string)  [unwired: 14 in]
          }
          frame "Set: Lockin Channel Amplitude" {
            n133 = Unbundle By Name(w394) -> ("Instruments.Lockin"=w390:refnum<class "Instrument.Lockin.lvclass">)
            n134 = flat-sequence {
              tunnel: w393 -> [_]
              tunnel: [0 ("Target Field (T)")] -> w392
              tunnel: [0.0 ("Target Rate (T/min)")] -> w391
              frame #0 {
              }
            }
            n135 = call <userlib>:"setAO_Amp.vi"("error in (no error)"=w389, "Amplitude (V)"=w391, "AO Channel"=w392, "Instrument.Lockin in"=w390) -> ("error out"=w395:errorcluster)  [unwired: 6 in, 1 out]
            n136 = call <vilib>:"Add State(s) to Queue__jki_lib_state_machine.vi"("State(s) in (\"\")"=w398) -> ("States Out"=w397:string)  [unwired: 14 in]
          }
          frame "Set: Lockin Channel Frequency" {
            n137 = Unbundle By Name(w406) -> ("Instruments.Lockin"=w402:refnum<class "Instrument.Lockin.lvclass">)
            n138 = flat-sequence {
              tunnel: w405 -> [_]
              tunnel: [0 ("Target Field (T)")] -> w404
              tunnel: [0.0 ("Target Rate (T/min)")] -> w403
              frame #0 {
              }
            }
            n139 = call <userlib>:"setAO_f.vi"("error in (no error)"=w401, "Frequency (Hz)"=w403, "AO Channel"=w404, "Instrument.Lockin in"=w402) -> ("error out"=w407:errorcluster)  [unwired: 6 in, 1 out]
            n140 = call <vilib>:"Add State(s) to Queue__jki_lib_state_machine.vi"("State(s) in (\"\")"=w410) -> ("States Out"=w409:string)  [unwired: 14 in]
          }
          frame "Set: Lockin Channel Phase" {
            n141 = Unbundle By Name(w418) -> ("Instruments.Lockin"=w414:refnum<class "Instrument.Lockin.lvclass">)
            n142 = flat-sequence {
              tunnel: w417 -> [_]
              tunnel: [0 ("Target Field (T)")] -> w416
              tunnel: [0.0 ("Target Rate (T/min)")] -> w415
              frame #0 {
              }
            }
            n143 = call <userlib>:"setAO_phi.vi"("error in (no error)"=w413, "Phase (°)"=w415, "AO Channel"=w416, "Instrument.Lockin in"=w414) -> ("error out"=w419:errorcluster)  [unwired: 6 in, 1 out]
            n144 = call <vilib>:"Add State(s) to Queue__jki_lib_state_machine.vi"("State(s) in (\"\")"=w422) -> ("States Out"=w421:string)  [unwired: 14 in]
          }
          frame "Set: Lockin Channel Function" {
            n145 = Unbundle By Name(w430) -> ("Instruments.Lockin"=w426:refnum<class "Instrument.Lockin.lvclass">)
            n146 = flat-sequence {
              tunnel: w429 -> [_]
              tunnel: [0 ("Target Field (T)")] -> w428
              tunnel: [0.0 ("Target Rate (T/min)")] -> w427
              frame #0 {
              }
            }
            n147 = call <userlib>:"setAO_function.vi"("error in (no error)"=w425, "Function"=w427, "AO Channel"=w428, "Instrument.Lockin in"=w426) -> ("error out"=w431:errorcluster)  [unwired: 6 in, 1 out]
            n148 = call <vilib>:"Add State(s) to Queue__jki_lib_state_machine.vi"("State(s) in (\"\")"=w434) -> ("States Out"=w433:string)  [unwired: 14 in]
          }
          frame "---------- Lockin Sweep ----------" {
            n149 = call <vilib>:"Add State(s) to Queue__jki_lib_state_machine.vi"("State(s) in (\"\")"=w441) -> ("States Out"=w440:string)  [unwired: 14 in]
          }
          frame "Lockin Sweep: Configure" {
            n150 = Unbundle By Name(w446) -> ("Instruments.Lockin"=w445:refnum<class "Instrument.Lockin.lvclass">)
            n151 = call <userlib>:"setSweepConfiguration.vi"("error in (no error)"=w444, "Configure Sweep"=T6 {"Sweep Time (s)"=0.0, "Initial Wait (s)"=0.0, "Return to Start"=FALSE, "Channels"=[]}, "Instrument.Lockin in"=w445) -> ("error out"=w443:errorcluster)  [unwired: 7 in, 1 out]
            n152 = call <vilib>:"Add State(s) to Queue__jki_lib_state_machine.vi"("State(s) in (\"\")"=w449) -> ("States Out"=w448:string)  [unwired: 14 in]
          }
          frame "Lockin Sweep: Start" {
            n153 = Unbundle By Name(w455) -> ("Instruments.Lockin"=w454:refnum<class "Instrument.Lockin.lvclass">)
            n154 = call <userlib>:"startSweep.vi"("error in (no error)"=w453, "Instrument.Lockin in"=w454) -> ("error out"=w451:errorcluster, "Instrument.Lockin out"=w452:refnum<class "Instrument.Lockin.lvclass">)  [unwired: 8 in]
            n155 = call <userlib>:"waitStatusSweepingStarted.vi"("error in (no error)"=w451, "Instrument.Lockin in"=w452) -> ("error out"=w450:errorcluster)  [unwired: 8 in, 1 out]
            n156 = call <vilib>:"Add State(s) to Queue__jki_lib_state_machine.vi"("State(s) in (\"\")"=w458) -> ("States Out"=w457:string)  [unwired: 14 in]
          }
          frame "Lockin Sweep: Stop" {
            n157 = Unbundle By Name(w464) -> ("Instruments.Lockin"=w463:refnum<class "Instrument.Lockin.lvclass">)
            n158 = call <userlib>:"stopSweep.vi"("error in (no error)"=w462, "Instrument.Lockin in"=w463) -> ("error out"=w460:errorcluster, "Instrument.Lockin out"=w461:refnum<class "Instrument.Lockin.lvclass">)  [unwired: 8 in]
            n159 = call <userlib>:"waitStatusSweepingStopped.vi"("error in (no error)"=w460, "Instrument.Lockin in"=w461) -> ("error out"=w459:errorcluster)  [unwired: 8 in, 1 out]
            n160 = call <vilib>:"Add State(s) to Queue__jki_lib_state_machine.vi"("State(s) in (\"\")"=w467) -> ("States Out"=w466:string)  [unwired: 14 in]
          }
          frame "Lockin Sweep: Status" {
            # "#todo\ndo stuff?"
            n161 = Unbundle By Name(w472) -> ("Instruments.Lockin"=w471:refnum<class "Instrument.Lockin.lvclass">)
            n162 = call <userlib>:"getStatus.vi"("error in (no error)"=w470, "Instrument.Lockin"=w471) -> ("error out"=w469:errorcluster, "Status"=w468:T15)  [unwired: 7 in, 1 out]
            n163 = case shown="\"idle\", Default" w468 {
              frame "idle", Default {
              }
              frame "created" {
              }
              frame "started" {
              }
              frame "stopped" {
              }
              frame "sweeping" {
              }
            }
            n164 = call <vilib>:"Add State(s) to Queue__jki_lib_state_machine.vi"("State(s) in (\"\")"=w475) -> ("States Out"=w474:string)  [unwired: 14 in]
          }
          frame "---------- Get ----------" {
            n165 = call <vilib>:"Add State(s) to Queue__jki_lib_state_machine.vi"("State(s) in (\"\")"=w480) -> ("States Out"=w479:string)  [unwired: 14 in]
          }
          frame "Get: Time" {
            n166 = Get Date/Time In Seconds() -> (seconds since 1Jan1904=w481:timestamp)
            n167 = To Double Precision Float(number=w481) -> (double precision float=w483:dbl)
            n168 = Bundle By Name(cluster=w485, "value"=w483) -> (w484:T11)
            n169 = call <vilib>:"Add State(s) to Queue__jki_lib_state_machine.vi"("State(s) in (\"\")"=w488) -> ("States Out"=w487:string)  [unwired: 14 in]
          }
          frame "Get: Temperature" {
            n170 = Unbundle By Name(w491) -> ("Instruments.Temperature"=w490:refnum<class "Instrument.Cryostat.lvclass">)
            n171 = call-dynamic "Get Temperature.vi"("error in (no error)"=w489, "Instrument.Cryostat in"=w490) -> ("error out"=w493:errorcluster, "Temperature (K)"=w492:dbl)  [unwired: 5 in, 3 out]
            n172 = Bundle By Name(cluster=w491, "value"=w492) -> (w494:T11)
            n173 = call <vilib>:"Add State(s) to Queue__jki_lib_state_machine.vi"("State(s) in (\"\")"=w497) -> ("States Out"=w496:string)  [unwired: 14 in]
          }
          frame "Get: Magnet" {
            n174 = Unbundle By Name(w500) -> ("Instruments.Magnet"=w499:refnum<class "Instrument.Cryostat.lvclass">)
            n175 = call-dynamic "Get Magnet.vi"("error in (no error)"=w498, "Instrument.Cryostat in"=w499) -> ("error out"=w502:errorcluster, "B Field (T)"=w501:dbl)  [unwired: 5 in, 3 out]
            n176 = Bundle By Name(cluster=w500, "value"=w501) -> (w503:T11)
            n177 = call <vilib>:"Add State(s) to Queue__jki_lib_state_machine.vi"("State(s) in (\"\")"=w506) -> ("States Out"=w505:string)  [unwired: 14 in]
          }
          frame "Get: Capacitance" {
            n178 = Unbundle By Name(w509) -> ("Instruments.Capacitance Bridge"=w508:refnum<class "Instrument.CBridge.lvclass">)
            n179 = call-dynamic "Get Capacitance.vi"("error in (no error)"=w507, "Instrument.CBridge in"=w508) -> ("error out"=w511:errorcluster, "Capacitance (pF)"=w510:dbl)  [unwired: 7 in, 1 out]
            n180 = Bundle By Name(cluster=w509, "value"=w510) -> (w512:T11)
            n181 = call <vilib>:"Add State(s) to Queue__jki_lib_state_machine.vi"("State(s) in (\"\")"=w515) -> ("States Out"=w514:string)  [unwired: 14 in]
          }
          frame "Get: Strain" {
            n182 = Unbundle By Name(w518) -> ("Instruments.Strain Cell"=w517:refnum<class "Instrument.Strain.lvclass">)
            n183 = call-dynamic "Get Strain.vi"("error in (no error)"=w516, "Instrument.Strain in"=w517) -> ("error out"=w520:errorcluster, "Strain (V)"=w519:dbl)  [unwired: 7 in, 1 out]
            n184 = Bundle By Name(cluster=w518, "value"=w519) -> (w521:T11)
            n185 = call <vilib>:"Add State(s) to Queue__jki_lib_state_machine.vi"("State(s) in (\"\")"=w524) -> ("States Out"=w523:string)  [unwired: 14 in]
          }
          frame "Get: Delay" {
            n186 = Unbundle By Name(w527) -> ("Instruments.Delay Line"=w526:refnum<class "Instrument.DelayLine.lvclass">)
            n187 = call-dynamic "Get Delay.vi"("error in (no error)"=w525, "Instrument.Delay in"=w526) -> ("error out"=w529:errorcluster, "Delay (ps)"=w528:dbl)  [unwired: 6 in, 2 out]
            n188 = Bundle By Name(cluster=w527, "value"=w528) -> (w530:T11)
            n189 = call <vilib>:"Add State(s) to Queue__jki_lib_state_machine.vi"("State(s) in (\"\")"=w533) -> ("States Out"=w532:string)  [unwired: 14 in]
          }
          frame "Get: Lockin AO" {
            n190 = Unbundle By Name(w536) -> ("Instruments.Lockin"=w535:refnum<class "Instrument.Lockin.lvclass">)
            n191 = call <userlib>:"getAOwfm.vi"("error in (no error)"=w534, "Instrument.Lockin in"=w535) -> ("error out"=w538:errorcluster, "AO Waveforrm"=w537:waveform(dbl)[])  [unwired: 7 in, 1 out]
            n192 = Bundle By Name(cluster=w536, "value"=w537) -> (w539:T11)
            n193 = call <vilib>:"Add State(s) to Queue__jki_lib_state_machine.vi"("State(s) in (\"\")"=w542) -> ("States Out"=w541:string)  [unwired: 14 in]
          }
          frame "Get: Lockin AI" {
            n194 = Unbundle By Name(w545) -> ("Instruments.Lockin"=w544:refnum<class "Instrument.Lockin.lvclass">)
            n195 = call <userlib>:"getAIwfm.vi"("error in (no error)"=w543, "Instrument.Lockin in"=w544) -> ("error out"=w547:errorcluster, "AI Waveform"=w546:waveform(dbl)[])  [unwired: 7 in, 1 out]
            n196 = Bundle By Name(cluster=w545, "value"=w546) -> (w548:T11)
            n197 = call <vilib>:"Add State(s) to Queue__jki_lib_state_machine.vi"("State(s) in (\"\")"=w551) -> ("States Out"=w550:string)  [unwired: 14 in]
          }
          frame "Get: Lockin Result" {
            n198 = Unbundle By Name(w554) -> ("Instruments.Lockin"=w553:refnum<class "Instrument.Lockin.lvclass">)
            n199 = call <userlib>:"getResults.vi"("error in (no error)"=w552, "Instrument.Lockin in"=w553) -> ("error out"=w556:errorcluster, "Results (Dictionary)"=w555:cluster{"key":string, "value":dbl}[])  [unwired: 6 in, 2 out]
            n200 = Bundle By Name(cluster=w554, "value"=w555) -> (w557:T11)
            n201 = call <vilib>:"Add State(s) to Queue__jki_lib_state_machine.vi"("State(s) in (\"\")"=w560) -> ("States Out"=w559:string)  [unwired: 14 in]
          }
        }
      }
    }
    frame Error {
    }
  }
  n202 = call-parent "Process.vi"("error in"=w5, "SMO"=w4) -> ("error out"=w2:errorcluster, "SMO out"=→"Transport out":refnum<class "SMO.Transport.lvclass">)  [unwired: 8 in]
  n203 = Merge Errors(w2, w1) -> (→"error out":errorcluster)
